vi "SCA_count.vi"() -> (0 "Acnt":i32)   [LabVIEW 2014]
panel:
  out "coincnt":i32
  out "Bcnt":i32
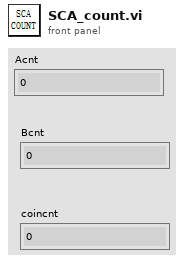
[diagram p1: front panel]
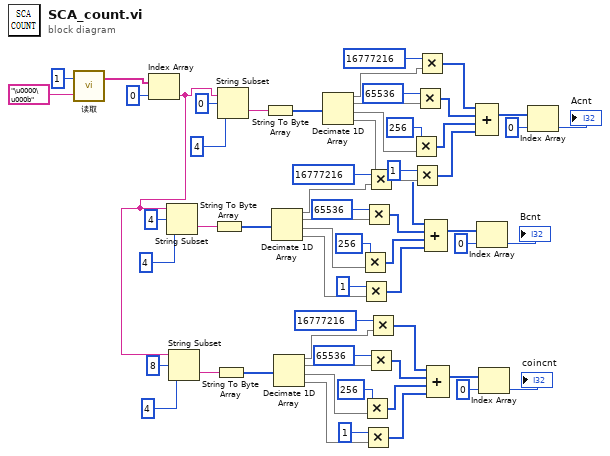
[diagram p0: block diagram]
diagram:
  n1 = call "读取.vi"("命令"="\u0000\u000b", "帧数"=1) -> ("数组"=w40:string[])  [unwired: 1 out]
  n2 = Index Array(array=w40, index=0 ("索引")) -> (element=w1:string)
  n3 = String Subset(string=w1, offset (0)=4 ("偏移量(0)"), length (rest)=4 ("长度（剩余）")) -> (substring=w25:string)
  n4 = String Subset(string=w1, offset (0)=8 ("偏移量(0)"), length (rest)=4 ("长度（剩余）")) -> (substring=w6:string)
  n5 = String To Byte Array(string=w25) -> (unsigned byte array=w24:u8[])
  n6 = String To Byte Array(string=w6) -> (unsigned byte array=w5:u8[])
  n7 = String Subset(string=w1, offset (0)=0 ("偏移量(0)"), length (rest)=4 ("长度（剩余）")) -> (substring=w45:string)
  n8 = String To Byte Array(string=w45) -> (unsigned byte array=w44:u8[])
  n9 = Decimate 1D Array(w24) -> (w26:u8[], w27:u8[], w37:u8[], w36:u8[])
  n10 = Decimate 1D Array(w5) -> (w7:u8[], w8:u8[], w18:u8[], w17:u8[])
  n11 = Decimate 1D Array(w44) -> (w46:u8[], w47:u8[], w57:u8[], w56:u8[])
  n12 = Multiply(x=256, y=w37) -> (x*y=w32:i32[])
  n13 = Multiply(x=1, y=w36) -> (x*y=w33:i32[])
  n14 = Multiply(x=256, y=w18) -> (x*y=w13:i32[])
  n15 = Multiply(x=1, y=w17) -> (x*y=w14:i32[])
  n16 = Multiply(x=65536, y=w27) -> (x*y=w29:i32[])
  n17 = Multiply(x=16777216, y=w26) -> (x*y=w28:i32[])
  n18 = Multiply(x=65536, y=w8) -> (x*y=w10:i32[])
  n19 = Multiply(x=16777216, y=w7) -> (x*y=w9:i32[])
  n20 = Multiply(x=256, y=w57) -> (x*y=w52:i32[])
  n21 = Multiply(x=1, y=w56) -> (x*y=w53:i32[])
  n22 = Multiply(x=65536, y=w47) -> (x*y=w49:i32[])
  n23 = Multiply(x=16777216, y=w46) -> (x*y=w48:i32[])
  n24 = Compound Arithmetic op=ADD(w28, w29, w32, w33) -> (w23:i32[])
  n25 = Compound Arithmetic op=ADD(w9, w10, w13, w14) -> (w4:i32[])
  n26 = Compound Arithmetic op=ADD(w48, w49, w52, w53) -> (w43:i32[])
  n27 = Index Array(array=w23, index=0 ("索引")) -> (element=→"Bcnt":i32)
  n28 = Index Array(array=w4, index=0 ("索引")) -> (element=→"coincnt":i32)
  n29 = Index Array(array=w43, index=0 ("索引")) -> (element=→"Acnt":i32)
